vi "Confluence API Utility.vi"() -> ()   [LabVIEW 2023]
uses:
  <userlib>/_PetranWay/LabVIEW Confluence API/Source/Confluence/Page/Page.lvclass/Page.ctl
  <userlib>/_PetranWay/LabVIEW Confluence API/Source/Confluence/Page/Accessors/Read storage value.vi
  <userlib>/_PetranWay/LabVIEW Confluence API/Source/Confluence/Page/Accessors/Read storage value.vi/24cc900c-cd5f-46ff-be78-0781b543e64e.vi
  <userlib>/_PetranWay/LabVIEW Confluence API/Source/Cloud/Confluence Cloud/Confluence Cloud.lvclass
  C:/Program Files/National Instruments/LabVIEW 2023/user.lib/_PetranWay/LabVIEW Confluence API/Source/Confluence/Confluence Connection/Confluence.lvclass
  <userlib>/_PetranWay/LabVIEW Confluence API/Source/Data Center/Confluence Data Center/Confluence Data Center.lvclass
  <userlib>/_PetranWay/LabVIEW Confluence API/Source/Cloud/Confluence Cloud/API/Construct Confluence Cloud From Cache.vi
  <userlib>/_PetranWay/LabVIEW Confluence API/Source/Data Center/Confluence Data Center/API/Construct Confluence Data Center From Cache.vi
  <vilib>/JDP Science/JSONtext/JSON text to Variant.vi
  <vilib>/JDP Science/JSONtext/LVClass Serializer/JSONtext LVClass Serializer.lvclass
  <userlib>/_PetranWay/LabVIEW Confluence API/Source/Confluence/Confluence Connection/Confluence.lvclass
  <userlib>/_PetranWay/LabVIEW Confluence API/Source/Confluence/Page/Page.lvclass
  <userlib>/_PetranWay/LabVIEW Confluence API/Source/Confluence/iConfluence/iConfluence.lvclass
panel:
  out "Error Out":errorcluster
  in  "Action":enum32{"Get Content", "Delete Child Pages"}(tab)
  out "Page Content":string
  out "Number of Pages Removed":u32
  in  "Connection":enum32{"Cloud", "Data Center"}(tab)
  in  "Email Address":string
  in  "Organization Name":string caption="Organization Name (https://[Organization Name].atlassian.net]"
  in  "Server URL":string
  in  "Top Page ID":string
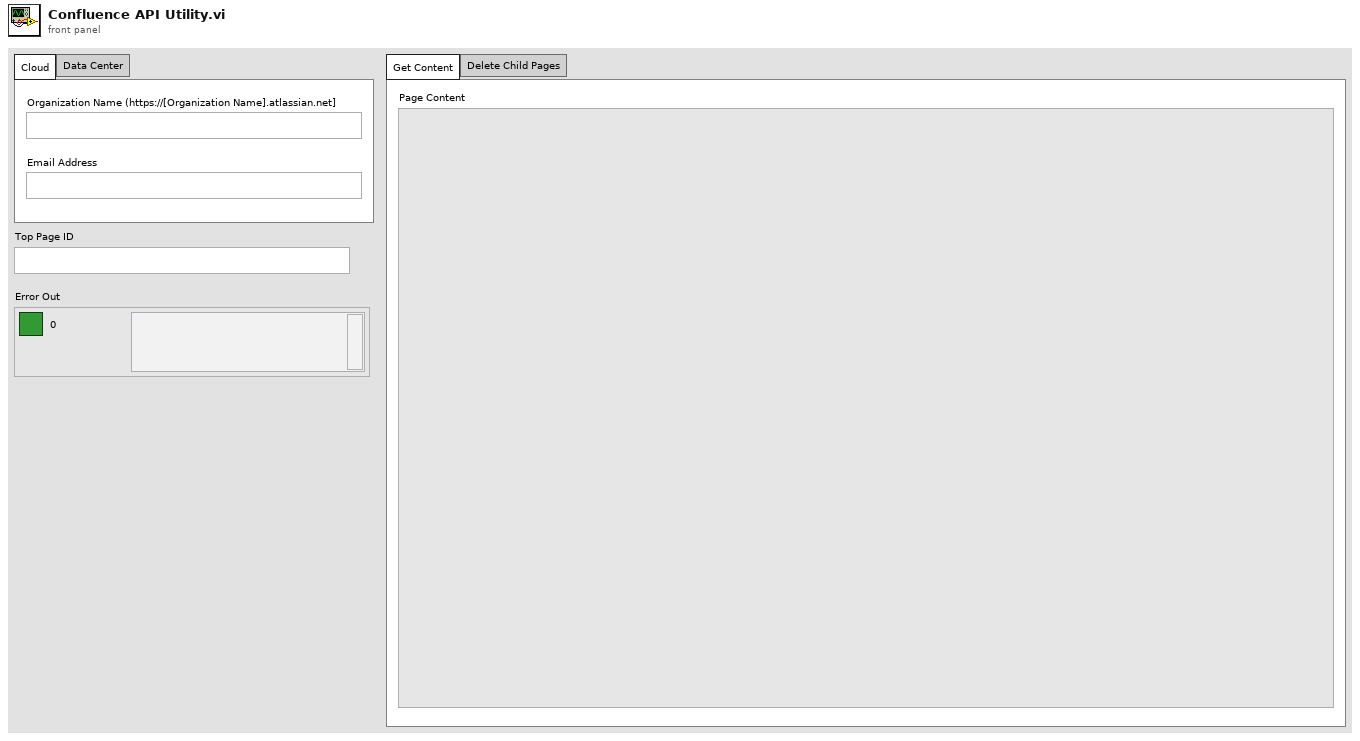
[diagram p1: front panel]
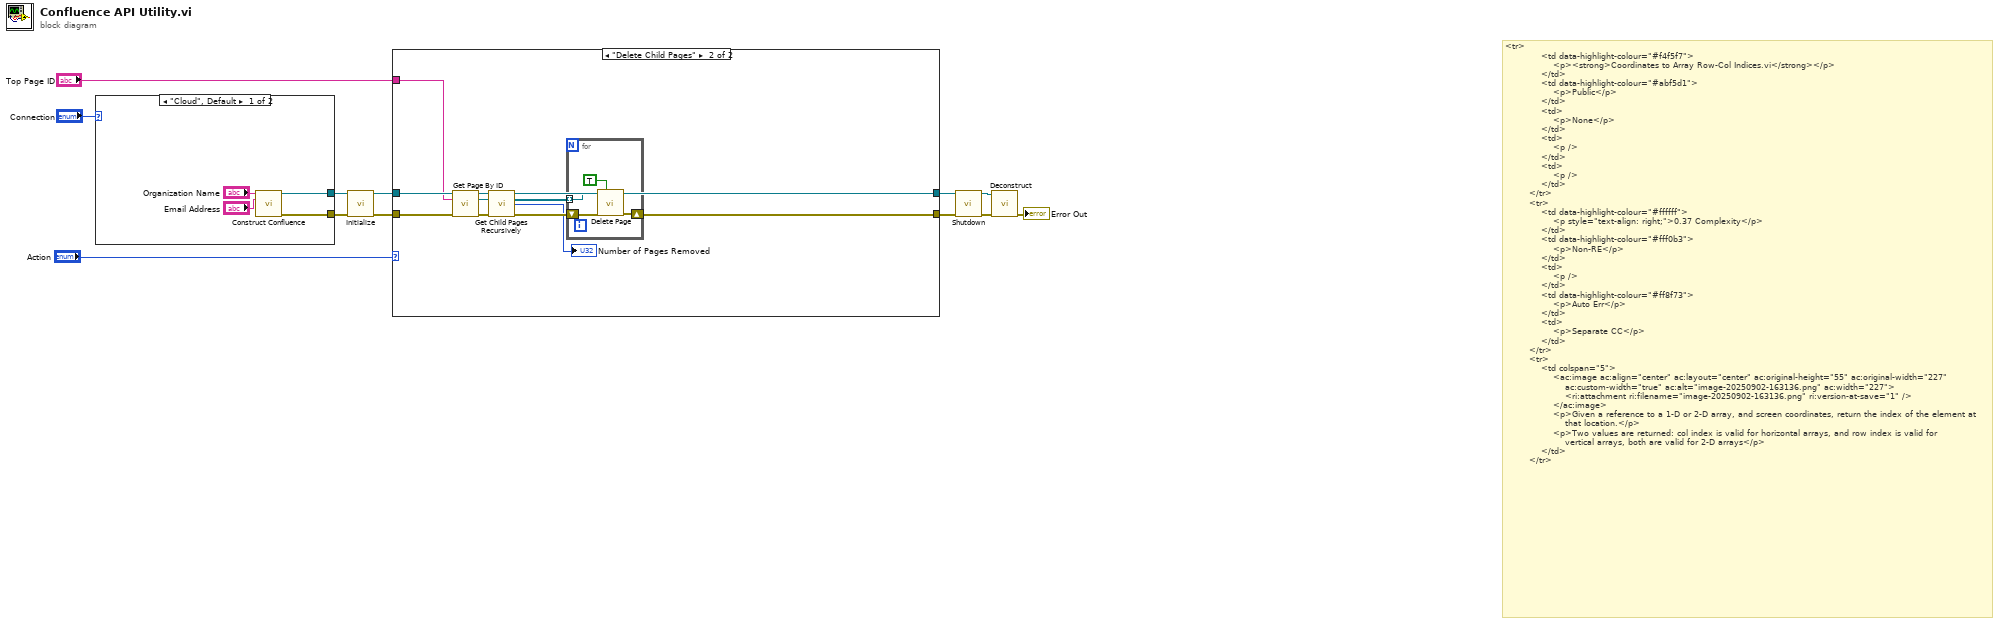
[diagram p0: block diagram]
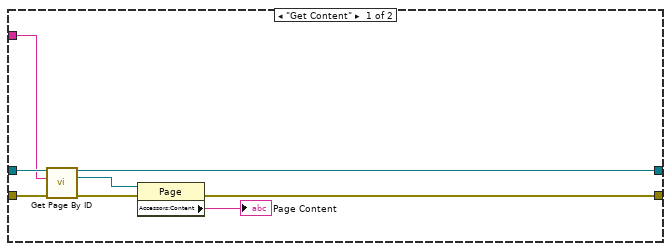
[diagram p2: hidden frame]
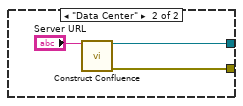
[diagram p3: hidden frame]
diagram:
  # "<tr>\n            <td data-highlight-colour=\"#f4f5f7\">\n                <p><strong>Coordinates to Array Row-Col Indices.vi</strong></p>\n            </td>\n            <td data-highlight-colour=\"#abf5d1\">\n                <p>Public</p>\n            </td>\n            <td>\n                <p>None</p>\n            </td>\n            <td>\n                <p />\n            </td>\n            <td>\n                <p />\n            </td>\n        </tr>\n        <tr>\n            <td data-highlight-colour=\"#ffffff\">\n                <p style=\"text-align: right;\">0.37 Complexity</p>\n            </td>\n            <td data-highlight-colour=\"#fff0b3\">\n                <p>Non-RE</p>\n            </td>\n            <td>\n                <p />\n            </td>\n            <td data-highlight-colour=\"#ff8f73\">\n                <p>Auto Err</p>\n            </td>\n            <td>\n                <p>Separate CC</p>\n            </td>\n        </tr>\n        <tr>\n            <td colspan=\"5\">\n                <ac:image ac:align=\"center\" ac:layout=\"center\" ac:original-height=\"55\" ac:original-width=\"227\"\n                    ac:custom-width=\"true\" ac:alt=\"image-20250902-163136.png\" ac:width=\"227\">\n                    <ri:attachment ri:filename=\"image-20250902-163136.png\" ri:version-at-save=\"1\" />\n                </ac:image>\n                <p>Given a reference to a 1-D or 2-D array, and screen coordinates, return the index of the element at\n                    that location.</p>\n                <p>Two values are returned: col index is valid for horizontal arrays, and row index is valid for\n                    vertical arrays, both are valid for 2-D arrays</p>\n            </td>\n        </tr>"
  n1 = case shown="\"Cloud\", Default" "Connection" {
    tunnel: [w15 w18] -> w9
    tunnel: [w16 w17] -> w8
    frame "Cloud", Default {
      n2 = call-poly <userlib>:"Construct Confluence.vi"("Organization Name (https://[Organization Name].atlassian.net]"="Organization Name", "Email Address"="Email Address") -> ("Confluence Cloud out"=w15:refnum<class "Confluence Cloud.lvclass">, "error out"=w16:errorcluster)  [unwired: 10 in, 2 out]
    }
    frame "Data Center" {
      n3 = call-poly <userlib>:"Construct Confluence.vi"("Server URL"="Server URL") -> ("Confluence Data Center out"=w18:refnum<class "Confluence Data Center.lvclass">, "error out"=w17:errorcluster)  [unwired: 11 in, 2 out]
    }
  }
  n4 = call-dynamic "Initialize.vi"("Confluence in"=w9, "error in (no error)"=w8) -> ("Confluence out"=w6:refnum<class "Confluence.lvclass">, "error out"=w5:errorcluster)  [unwired: 12 in]
  n5 = case shown="\"Delete Child Pages\"" "Action" {
    tunnel: w6 -> [w27 w33]
    tunnel: w5 -> [w26 w34]
    tunnel: "Top Page ID" -> [w25 w32]
    tunnel: [w21 w28] -> w3
    tunnel: [w20 w30] -> w1
    frame "Get Content" {
      n6 = call-dynamic "Get Page By ID.vi"("Confluence Connection in"=w27, "ID"=w25, "error in (no error)"=w26) -> ("Atlassian Connection out"=w20:refnum<class "Confluence.lvclass">, "Page out"=w23:refnum<class "Page.lvclass">, "error out"=w24:errorcluster)  [unwired: 9 in, 1 out]
      n7 = property class="Page"(reference=w23, error in=w24) -> (error out=w21:errorcluster, "Accessors:Content"=→"Page Content":string)  [unwired: 1 out]
    }
    frame "Delete Child Pages" {
      n8 = call-dynamic "Get Page By ID.vi"("Confluence Connection in"=w33, "ID"=w32, "error in (no error)"=w34) -> ("Atlassian Connection out"=w37:refnum<class "Confluence.lvclass">, "Page out"=w35:refnum<class "Page.lvclass">, "error out"=w36:errorcluster)  [unwired: 9 in, 1 out]
      n9 = call-dynamic "Get Child Pages Recursively.vi"("Confluence in"=w37, "Page"=w35, "error in (no error)"=w36) -> ("Confluence out"=w30:refnum<class "Confluence.lvclass">, "Child Pages"=w38:refnum<class "Page.lvclass">[], "Number of pages"=→"Number of Pages Removed":u32, "error out"=w31:errorcluster)  [unwired: 9 in]
      n10 = for {
        tunnel: w38 -> [w42] mode=indexing
        shift-right: [w39] -> w28
        shift-left: w31 -> [w40]
        n11 = call-dynamic "Delete Page.vi"("Page"=w42, "Resursive Delete"=TRUE, "error in (no error)"=w40) -> ("error out"=w39:errorcluster)  [unwired: 12 in]
      }
    }
  }
  n12 = call-dynamic "Shutdown.vi"("Confluence in"=w1, "error in (no error)"=w3) -> ("Confluence out"=w12:refnum<class "Confluence.lvclass">, "error out"=w11:errorcluster)  [unwired: 12 in]
  n13 = call-dynamic "Deconstruct.vi"("error in (no error)"=w11, "Confluence in"=w12) -> ("error out"=→"Error Out":errorcluster)  [unwired: 9 in]
